vi "EstimateErrors.vi"(7 "Pose0 (X, Y, Theta)":dbl[](array[numeric])=[0.0, 0.0, 0.0], 8 "Circle variables errors":T4={"punktDistSquare"=[0.0, 0.07564773182654234, 0.07557311216319511, 0.07578803616247684, 0.07567014980458597, 0.07535518316388122, 0.0757185080544904, 0.07334892874492238, 0.07585576670877042, 0.07541545264649341, 0.07457142815247282, 0.0720824805087417, 0.06961575822916764, 0.06683871762791828, 0.0630284017195026, 0.059082964720348206, 0.05355458998235239, 0.05045461701579379, 0.04470630680818257, 0.03964739483907835, 0.03453253618111823, 0.02904994482413108, 0.023688402162769955, 0.01892536585845739, 0.014215766563588304, 0.010250329125772036, 0.006818695465891372, 0.003943465844516061, 0.0020809448605467406, 0.0005220835606117719, 1.2383649131457327e-05, 0.0003390725932862521, 0.001540945833685875, 0.0035195264049144095, 0.0060279610827917935, 0.008761138637480492, 0.012367610332300055, 0.01627487568319867, 0.020308106515570287, 0.024594534493235544, 0.028943415071940114, 0.03341115784396496, 0.037285381727813045, 0.04126201164451483, 0.045079825351421264, 0.04914306964453862, 0.0514613643484263, 0.05428534924131425, 0.05625555787449453, 0.05657242294416296, 0.05651616674073519, 0.055951366501415835, 0.054616628689924826, 0.05239466959604635, 0.05005043029476607, 0.04679005433056029, 0.042887475499745156, 0.0387519129163008, 0.0336280677551115, 0.02966200797528215, 0.025266909215039494, 0.02072471019982025, 0.016797122005156952, 0.012291220019395255, 0.008810089263448142, 0.00567593978669209, 0.003349003924343437, 0.0014861104439980038, 0.00043833446681027654, 3.9034156999441e-06, 0.00010421819224661581, 0.0006618229911799063, 0.0013807697493980796, 0.002218800940383718, 0.0032733224891644593, 0.004574912694052916, 0.005507405786350822, 0.006413953108626536, 0.007416403488251084, 0.007799062706470956, 0.007900128314354375, 0.007695822505959842, 0.007105496206833856, 0.006394343915694971, 0.005455973268666394, 0.004255972699592567, 0.0029149765928852653, 0.001966512463123503, 0.0009603861261508478, 0.0002841530345349927, 8.156616622773978e-06, 0.0004068005644318846, 0.0016844789753319045, 0.0036816048553430366, 0.007279831590487791, 0.01211319395311253, 0.018235687252944322, 0.025815049718371556, 0.03477395530382172, 0.04594658715803277, 0.05940579170402822, 0.07195291174212014, 0.08883550205094089, 0.10614135307735591, 0.12610066821536306, 0.14715212125088853, 0.1717623938366619, 0.1969362684280186, 0.2248206059063523, 0.00012726523840876527, 0.00012280960585971167, 3.0014150177905496e-05, 0.00044221993068126696, 0.0026874041910711797, 0.015825445797725355, 0.04630193476148654, 0.07938556772924259, 0.09054009974589632], "X travelled"=[0.0, 1.2695120888079892, 1.2692312255127836, 1.2694654526261373, 1.2692477473907526, 1.2691017901849175, 1.2696542995423077, 1.2571532097357658, 1.2387575500923158, 1.216600111019282, 1.192192947184398, 1.167405514173482, 1.1413899163623515, 1.1150560373224825, 1.0874230986410096, 1.0638480524217664, 1.0398001723629628, 1.0146852541804219, 0.9923351075893959, 0.9685827340265091, 0.9432369365366903, 0.9170882628506359, 0.8917289878071746, 0.8686417555900694, 0.8439669533526823, 0.8199720439623648, 0.7956956103849276, 0.7720631355922368, 0.7489369018852821, 0.7237191149505686, 0.6992024917565707, 0.6747186374632433, 0.6503530875312046, 0.6252720411425005, 0.6017948697201847, 0.5788637764853476, 0.5550605203636303, 0.5312645310848891, 0.5077586901078085, 0.48151679846144435, 0.45674499934516527, 0.42976239752787115, 0.4047903368931877, 0.37800013536527355, 0.353457975553972, 0.321633095547316, 0.29685338790972066, 0.26621470497176003, 0.23640735895233098, 0.2046386706338113, 0.1757786957333123, 0.14453904740116533, 0.11588563434771729, 0.08443371862104453, 0.0561871655388403, 0.026630408440516815, -0.00314924246510887, -0.030887936500388236, -0.06070435130947068, -0.08903243103192268, -0.11216261518885712, -0.1391091582848538, -0.1654116103393078, -0.19101893289595676, -0.2152215884303818, -0.23994715714337814, -0.265062748085184, -0.28831589903809757, -0.3118249838362658, -0.33485539410810033, -0.35943310881112206, -0.38168948393512264, -0.4051724359779647, -0.4317614148947837, -0.4544812996670769, -0.47653452740076285, -0.5026117792886527, -0.5258360330870897, -0.5507479667209695, -0.5766609558687512, -0.6002049112959483, -0.6265170935089266, -0.6519533931466335, -0.6785689453981383, -0.7034682073883944, -0.7278750721133671, -0.757191632268316, -0.7841548638522253, -0.8126279679466061, -0.8402415342318459, -0.8700108849679966, -0.9003257232864297, -0.9319275221467972, -0.9601668175409852, -0.9911787612489938, -1.0225070550459336, -1.0530758282656856, -1.0832624494521472, -1.113028095420975, -1.1441614405859464, -1.1746594514768973, -1.2021620653253586, -1.231726719500456, -1.2590665391582947, -1.2879782803828206, -1.3153404019292236, -1.3437046572531026, -1.3710522627012873, -1.398141963895538, -0.9209240462698031, -0.9210089892186536, -0.9041765205215978, -0.8566600027574827, -0.7504973452310854, -0.6062134912938122, -0.43036863858250807, -0.2550474545013706, -0.12907825402937256], "Y travelled"=[0.0, 1.2997835570201033, 1.299918266998385, 1.2995290477144008, 1.2997419532092793, 1.3003139694205859, 1.2996536097512235, 1.3039920884611322, 1.2994203274600276, 1.3002295297448985, 1.3017859072669729, 1.3063977887786817, 1.311048954293369, 1.316389275617112, 1.3238759854456834, 1.33188115664532, 1.3435550315578317, 1.3503687265675801, 1.3635524859658168, 1.375893604914819, 1.3891951203545152, 1.4045990740324474, 1.421146766916605, 1.4375053137323193, 1.4558644369719869, 1.4738853501994724, 1.4925638161546586, 1.5123376556556292, 1.5295457563837995, 1.5523340107584074, 1.5719536798753582, 1.5935114583075545, 1.6143863909036604, 1.634504558758891, 1.6528717287556438, 1.6688520864593281, 1.6864617161758972, 1.7028457289160475, 1.7178066107992285, 1.732135219670476, 1.7454546164708304, 1.758131127043267, 1.7684545144678636, 1.7785136756666506, 1.7877191136549149, 1.7970948178568789, 1.8022807728780508, 1.808436129290746, 1.8126471307419418, 1.8133410693098495, 1.8132335115605274, 1.8120709817533533, 1.8092419191532152, 1.804468328920625, 1.7992945699811371, 1.7919075661447772, 1.7827107912063302, 1.7724991714524176, 1.7590423567427707, 1.7478950251350323, 1.734648646961109, 1.7196602851886198, 1.7053321558620678, 1.6866123399737936, 1.6696203858108163, 1.651108728261376, 1.6336564904406876, 1.6142896803462332, 1.5967434706070807, 1.5774676467398316, 1.559575053267482, 1.5380139222042355, 1.5202931680977338, 1.5020652392071476, 1.4831114145715987, 1.4640399847051702, 1.44633932925363, 1.4286940336279008, 1.4100473033558134, 1.3934713992454555, 1.3785351020910583, 1.3639032285078156, 1.3508931942803428, 1.3365341066050573, 1.3256050266509627, 1.3176014816898536, 1.306502275234161, 1.2953169075402846, 1.2876909060075314, 1.2797977569282104, 1.2749442960425688, 1.2696805567666585, 1.2664096698763037, 1.2639092252393325, 1.2643295206125267, 1.2646313441406596, 1.2662172911660277, 1.2693340306245853, 1.273250028069598, 1.2786250047164172, 1.2863436394563064, 1.2893514799759693, 1.2987257080431716, 1.307715372397717, 1.3171558179397458, 1.3274743163358067, 1.3405108730642281, 1.3523620445922784, 1.366490163526435, -0.6855341381820631, -0.6857707309878518, -0.7136948176982961, -0.8033890120521333, -0.9346796502513917, -1.106006471640569, -1.2607529582490453, -1.3395413306604762, -1.358591049628456]}, 9 "Pose (X, Y, Theta)":dbl[](array[numeric])=[0.0, 0.0, 0.0], 10 "Trajectory":T6={"X path"=array[1899 elements], "Y path"=array[1899 elements], "Theta path"=array[1899 elements]}, 11 "Clear Graph":bool) -> (0 "Circle variables errors out":T5={"punktDistSquare"=[0.0+0.0i, 0.07564773182654234+0.0i, 0.07557311216319511+0.0i, 0.07578803616247684+0.0i, 0.07567014980458597+0.0i, 0.07535518316388122+0.0i, 0.0757185080544904+0.0i, 0.07334892874492238+0.0i, 0.07585576670877042+0.0i, 0.07541545264649341+0.0i, 0.07457142815247282+0.0i, 0.0720824805087417+0.0i, 0.06961575822916764+0.0i, 0.06683871762791828+0.0i, 0.0630284017195026+0.0i, 0.059082964720348206+0.0i, 0.05355458998235239+0.0i, 0.05045461701579379+0.0i, 0.04470630680818257+0.0i, 0.03964739483907835+0.0i, 0.03453253618111823+0.0i, 0.02904994482413108+0.0i, 0.023688402162769955+0.0i, 0.01892536585845739+0.0i, 0.014215766563588304+0.0i, 0.010250329125772036+0.0i, 0.006818695465891372+0.0i, 0.003943465844516061+0.0i, 0.0020809448605467406+0.0i, 0.0005220835606117719+0.0i, 1.2383649131457327e-05+0.0i, 0.0003390725932862521+0.0i, 0.001540945833685875+0.0i, 0.0035195264049144095+0.0i, 0.0060279610827917935+0.0i, 0.008761138637480492+0.0i, 0.012367610332300055+0.0i, 0.01627487568319867+0.0i, 0.020308106515570287+0.0i, 0.024594534493235544+0.0i, 0.028943415071940114+0.0i, 0.03341115784396496+0.0i, 0.037285381727813045+0.0i, 0.04126201164451483+0.0i, 0.045079825351421264+0.0i, 0.04914306964453862+0.0i, 0.0514613643484263+0.0i, 0.05428534924131425+0.0i, 0.05625555787449453+0.0i, 0.05657242294416296+0.0i, 0.05651616674073519+0.0i, 0.055951366501415835+0.0i, 0.054616628689924826+0.0i, 0.05239466959604635+0.0i, 0.05005043029476607+0.0i, 0.04679005433056029+0.0i, 0.042887475499745156+0.0i, 0.0387519129163008+0.0i, 0.0336280677551115+0.0i, 0.02966200797528215+0.0i, 0.025266909215039494+0.0i, 0.02072471019982025+0.0i, 0.016797122005156952+0.0i, 0.012291220019395255+0.0i, 0.008810089263448142+0.0i, 0.00567593978669209+0.0i, 0.003349003924343437+0.0i, 0.0014861104439980038+0.0i, 0.00043833446681027654+0.0i, 3.9034156999441e-06+0.0i, 0.00010421819224661581+0.0i, 0.0006618229911799063+0.0i, 0.0013807697493980796+0.0i, 0.002218800940383718+0.0i, 0.0032733224891644593+0.0i, 0.004574912694052916+0.0i, 0.005507405786350822+0.0i, 0.006413953108626536+0.0i, 0.007416403488251084+0.0i, 0.007799062706470956+0.0i, 0.007900128314354375+0.0i, 0.007695822505959842+0.0i, 0.007105496206833856+0.0i, 0.006394343915694971+0.0i, 0.005455973268666394+0.0i, 0.004255972699592567+0.0i, 0.0029149765928852653+0.0i, 0.001966512463123503+0.0i, 0.0009603861261508478+0.0i, 0.0002841530345349927+0.0i, 8.156616622773978e-06+0.0i, 0.0004068005644318846+0.0i, 0.0016844789753319045+0.0i, 0.0036816048553430366+0.0i, 0.007279831590487791+0.0i, 0.01211319395311253+0.0i, 0.018235687252944322+0.0i, 0.025815049718371556+0.0i, 0.03477395530382172+0.0i, 0.04594658715803277+0.0i, 0.05940579170402822+0.0i, 0.07195291174212014+0.0i, 0.08883550205094089+0.0i, 0.10614135307735591+0.0i, 0.12610066821536306+0.0i, 0.14715212125088853+0.0i, 0.1717623938366619+0.0i, 0.1969362684280186+0.0i, 0.2248206059063523+0.0i, 0.00012726523840876527+0.0i, 0.00012280960585971167+0.0i, 3.0014150177905496e-05+0.0i, 0.00044221993068126696+0.0i, 0.0026874041910711797+0.0i, 0.015825445797725355+0.0i, 0.04630193476148654+0.0i, 0.07938556772924259+0.0i, 0.09054009974589632+0.0i, 0.0887296013230938+0.0i], "TrackX"=[0.0, 1.2695120888079892, 1.2692312255127836, 1.2694654526261373, 1.2692477473907526, 1.2691017901849175, 1.2696542995423077, 1.2571532097357658, 1.2387575500923158, 1.216600111019282, 1.192192947184398, 1.167405514173482, 1.1413899163623515, 1.1150560373224825, 1.0874230986410096, 1.0638480524217664, 1.0398001723629628, 1.0146852541804219, 0.9923351075893959, 0.9685827340265091, 0.9432369365366903, 0.9170882628506359, 0.8917289878071746, 0.8686417555900694, 0.8439669533526823, 0.8199720439623648, 0.7956956103849276, 0.7720631355922368, 0.7489369018852821, 0.7237191149505686, 0.6992024917565707, 0.6747186374632433, 0.6503530875312046, 0.6252720411425005, 0.6017948697201847, 0.5788637764853476, 0.5550605203636303, 0.5312645310848891, 0.5077586901078085, 0.48151679846144435, 0.45674499934516527, 0.42976239752787115, 0.4047903368931877, 0.37800013536527355, 0.353457975553972, 0.321633095547316, 0.29685338790972066, 0.26621470497176003, 0.23640735895233098, 0.2046386706338113, 0.1757786957333123, 0.14453904740116533, 0.11588563434771729, 0.08443371862104453, 0.0561871655388403, 0.026630408440516815, -0.00314924246510887, -0.030887936500388236, -0.06070435130947068, -0.08903243103192268, -0.11216261518885712, -0.1391091582848538, -0.1654116103393078, -0.19101893289595676, -0.2152215884303818, -0.23994715714337814, -0.265062748085184, -0.28831589903809757, -0.3118249838362658, -0.33485539410810033, -0.35943310881112206, -0.38168948393512264, -0.4051724359779647, -0.4317614148947837, -0.4544812996670769, -0.47653452740076285, -0.5026117792886527, -0.5258360330870897, -0.5507479667209695, -0.5766609558687512, -0.6002049112959483, -0.6265170935089266, -0.6519533931466335, -0.6785689453981383, -0.7034682073883944, -0.7278750721133671, -0.757191632268316, -0.7841548638522253, -0.8126279679466061, -0.8402415342318459, -0.8700108849679966, -0.9003257232864297, -0.9319275221467972, -0.9601668175409852, -0.9911787612489938, -1.0225070550459336, -1.0530758282656856, -1.0832624494521472, -1.113028095420975, -1.1441614405859464, -1.1746594514768973, -1.2021620653253586, -1.231726719500456, -1.2590665391582947, -1.2879782803828206, -1.3153404019292236, -1.3437046572531026, -1.3710522627012873, -1.398141963895538, -0.9209240462698031, -0.9210089892186536, -0.9041765205215978, -0.8566600027574827, -0.7504973452310854, -0.6062134912938122, -0.43036863858250807, -0.2550474545013706, -0.12907825402937256, -0.06378735155907347], "TrackY"=[0.0, 1.2997835570201033, 1.299918266998385, 1.2995290477144008, 1.2997419532092793, 1.3003139694205859, 1.2996536097512235, 1.3039920884611322, 1.2994203274600276, 1.3002295297448985, 1.3017859072669729, 1.3063977887786817, 1.311048954293369, 1.316389275617112, 1.3238759854456834, 1.33188115664532, 1.3435550315578317, 1.3503687265675801, 1.3635524859658168, 1.375893604914819, 1.3891951203545152, 1.4045990740324474, 1.421146766916605, 1.4375053137323193, 1.4558644369719869, 1.4738853501994724, 1.4925638161546586, 1.5123376556556292, 1.5295457563837995, 1.5523340107584074, 1.5719536798753582, 1.5935114583075545, 1.6143863909036604, 1.634504558758891, 1.6528717287556438, 1.6688520864593281, 1.6864617161758972, 1.7028457289160475, 1.7178066107992285, 1.732135219670476, 1.7454546164708304, 1.758131127043267, 1.7684545144678636, 1.7785136756666506, 1.7877191136549149, 1.7970948178568789, 1.8022807728780508, 1.808436129290746, 1.8126471307419418, 1.8133410693098495, 1.8132335115605274, 1.8120709817533533, 1.8092419191532152, 1.804468328920625, 1.7992945699811371, 1.7919075661447772, 1.7827107912063302, 1.7724991714524176, 1.7590423567427707, 1.7478950251350323, 1.734648646961109, 1.7196602851886198, 1.7053321558620678, 1.6866123399737936, 1.6696203858108163, 1.651108728261376, 1.6336564904406876, 1.6142896803462332, 1.5967434706070807, 1.5774676467398316, 1.559575053267482, 1.5380139222042355, 1.5202931680977338, 1.5020652392071476, 1.4831114145715987, 1.4640399847051702, 1.44633932925363, 1.4286940336279008, 1.4100473033558134, 1.3934713992454555, 1.3785351020910583, 1.3639032285078156, 1.3508931942803428, 1.3365341066050573, 1.3256050266509627, 1.3176014816898536, 1.306502275234161, 1.2953169075402846, 1.2876909060075314, 1.2797977569282104, 1.2749442960425688, 1.2696805567666585, 1.2664096698763037, 1.2639092252393325, 1.2643295206125267, 1.2646313441406596, 1.2662172911660277, 1.2693340306245853, 1.273250028069598, 1.2786250047164172, 1.2863436394563064, 1.2893514799759693, 1.2987257080431716, 1.307715372397717, 1.3171558179397458, 1.3274743163358067, 1.3405108730642281, 1.3523620445922784, 1.366490163526435, -0.6855341381820631, -0.6857707309878518, -0.7136948176982961, -0.8033890120521333, -0.9346796502513917, -1.106006471640569, -1.2607529582490453, -1.3395413306604762, -1.358591049628456, -1.3555183923263967]}, 1 "PathController inputs":T1, 2 "Truck data":T2={"RMS error"=0.0+0.0i, "DistanceAheadPointToTrajectory"=0.0+0.0i, "CurrentRefTheta"=0.04056520868612421, "CurrentThetaError"=-6.222088142143954, "DistanceCurrentPoseToTrajectory"=0.29787514384905267+0.0i, "MaximalDistance"=0.4741525133396978+0.0i}, 4 "Errors":cluster{"error_x":dbl, "error_y":dbl}, 5 "Plot variables":T3={"currentRefX"=-0.06646440361680006, "currentRefY"=-1.05765527827, "pointAhead"=[-0.06378735155907347, -1.3555183923263967], "TrackX"=[0.0, 1.2695120888079892, 1.2692312255127836, 1.2694654526261373, 1.2692477473907526, 1.2691017901849175, 1.2696542995423077, 1.2571532097357658, 1.2387575500923158, 1.216600111019282, 1.192192947184398, 1.167405514173482, 1.1413899163623515, 1.1150560373224825, 1.0874230986410096, 1.0638480524217664, 1.0398001723629628, 1.0146852541804219, 0.9923351075893959, 0.9685827340265091, 0.9432369365366903, 0.9170882628506359, 0.8917289878071746, 0.8686417555900694, 0.8439669533526823, 0.8199720439623648, 0.7956956103849276, 0.7720631355922368, 0.7489369018852821, 0.7237191149505686, 0.6992024917565707, 0.6747186374632433, 0.6503530875312046, 0.6252720411425005, 0.6017948697201847, 0.5788637764853476, 0.5550605203636303, 0.5312645310848891, 0.5077586901078085, 0.48151679846144435, 0.45674499934516527, 0.42976239752787115, 0.4047903368931877, 0.37800013536527355, 0.353457975553972, 0.321633095547316, 0.29685338790972066, 0.26621470497176003, 0.23640735895233098, 0.2046386706338113, 0.1757786957333123, 0.14453904740116533, 0.11588563434771729, 0.08443371862104453, 0.0561871655388403, 0.026630408440516815, -0.00314924246510887, -0.030887936500388236, -0.06070435130947068, -0.08903243103192268, -0.11216261518885712, -0.1391091582848538, -0.1654116103393078, -0.19101893289595676, -0.2152215884303818, -0.23994715714337814, -0.265062748085184, -0.28831589903809757, -0.3118249838362658, -0.33485539410810033, -0.35943310881112206, -0.38168948393512264, -0.4051724359779647, -0.4317614148947837, -0.4544812996670769, -0.47653452740076285, -0.5026117792886527, -0.5258360330870897, -0.5507479667209695, -0.5766609558687512, -0.6002049112959483, -0.6265170935089266, -0.6519533931466335, -0.6785689453981383, -0.7034682073883944, -0.7278750721133671, -0.757191632268316, -0.7841548638522253, -0.8126279679466061, -0.8402415342318459, -0.8700108849679966, -0.9003257232864297, -0.9319275221467972, -0.9601668175409852, -0.9911787612489938, -1.0225070550459336, -1.0530758282656856, -1.0832624494521472, -1.113028095420975, -1.1441614405859464, -1.1746594514768973, -1.2021620653253586, -1.231726719500456, -1.2590665391582947, -1.2879782803828206, -1.3153404019292236, -1.3437046572531026, -1.3710522627012873, -1.398141963895538, -0.9209240462698031, -0.9210089892186536, -0.9041765205215978, -0.8566600027574827, -0.7504973452310854, -0.6062134912938122, -0.43036863858250807, -0.2550474545013706, -0.12907825402937256, -0.06378735155907347], "TrackY"=[0.0, 1.2997835570201033, 1.299918266998385, 1.2995290477144008, 1.2997419532092793, 1.3003139694205859, 1.2996536097512235, 1.3039920884611322, 1.2994203274600276, 1.3002295297448985, 1.3017859072669729, 1.3063977887786817, 1.311048954293369, 1.316389275617112, 1.3238759854456834, 1.33188115664532, 1.3435550315578317, 1.3503687265675801, 1.3635524859658168, 1.375893604914819, 1.3891951203545152, 1.4045990740324474, 1.421146766916605, 1.4375053137323193, 1.4558644369719869, 1.4738853501994724, 1.4925638161546586, 1.5123376556556292, 1.5295457563837995, 1.5523340107584074, 1.5719536798753582, 1.5935114583075545, 1.6143863909036604, 1.634504558758891, 1.6528717287556438, 1.6688520864593281, 1.6864617161758972, 1.7028457289160475, 1.7178066107992285, 1.732135219670476, 1.7454546164708304, 1.758131127043267, 1.7684545144678636, 1.7785136756666506, 1.7877191136549149, 1.7970948178568789, 1.8022807728780508, 1.808436129290746, 1.8126471307419418, 1.8133410693098495, 1.8132335115605274, 1.8120709817533533, 1.8092419191532152, 1.804468328920625, 1.7992945699811371, 1.7919075661447772, 1.7827107912063302, 1.7724991714524176, 1.7590423567427707, 1.7478950251350323, 1.734648646961109, 1.7196602851886198, 1.7053321558620678, 1.6866123399737936, 1.6696203858108163, 1.651108728261376, 1.6336564904406876, 1.6142896803462332, 1.5967434706070807, 1.5774676467398316, 1.559575053267482, 1.5380139222042355, 1.5202931680977338, 1.5020652392071476, 1.4831114145715987, 1.4640399847051702, 1.44633932925363, 1.4286940336279008, 1.4100473033558134, 1.3934713992454555, 1.3785351020910583, 1.3639032285078156, 1.3508931942803428, 1.3365341066050573, 1.3256050266509627, 1.3176014816898536, 1.306502275234161, 1.2953169075402846, 1.2876909060075314, 1.2797977569282104, 1.2749442960425688, 1.2696805567666585, 1.2664096698763037, 1.2639092252393325, 1.2643295206125267, 1.2646313441406596, 1.2662172911660277, 1.2693340306245853, 1.273250028069598, 1.2786250047164172, 1.2863436394563064, 1.2893514799759693, 1.2987257080431716, 1.307715372397717, 1.3171558179397458, 1.3274743163358067, 1.3405108730642281, 1.3523620445922784, 1.366490163526435, -0.6855341381820631, -0.6857707309878518, -0.7136948176982961, -0.8033890120521333, -0.9346796502513917, -1.106006471640569, -1.2607529582490453, -1.3395413306604762, -1.358591049628456, -1.3555183923263967]})   [LabVIEW 2013]
uses:
  <vilib>/imath/engines/lvmath2/RunTimeEngine/ErrorHandling/NIMS_Finalize Error.vi
  <vilib>/imath/engines/lvmath2/RunTimeEngine/Managers/WorkSpace/UID Generator.vi
  <vilib>/imath/engines/lvmath2/RunTimeEngine/IndexRead/NIMS V(S).vi
  <instcachedir>/0/NIMS V(S)_0488751826AF41519A22953C041130DC.lvgen/NIMS V(S)_0488751826AF41519A22953C041130DC_000.vi
  <vilib>/imath/engines/lvmath2/RunTimeEngine/BuiltInFunctions/is_nan/NIMS_is_nan.vi
  <instcachedir>/0/NIMS_is_nan_BCCD798162CC49E3A8E57072444F6EB6.lvgen/NIMS_is_nan_BCCD798162CC49E3A8E57072444F6EB6_002.vi
  <vilib>/imathl/engines/lvmath/Functions/Error Handling/Create Error.vi
  <vilib>/imath/engines/lvmath2/RunTimeEngine/Managers/SymbolTable/Clear UID.vi
  <vilib>/imath/engines/lvmath2/RunTimeEngine/NodeEndStatement/NIMS_NodeEndStatement_Output.vi
  <instcachedir>/0/NIMS_NodeEndStatement_Output_53EC0D466D134D7ABD903AC30B43404B.lvgen/NIMS_NodeEndStatement_Output_53EC0D466D134D7ABD903AC30B43404B_010.vi
  <instcachedir>/0/NIMS_NodeEndStatement_Output_53EC0D466D134D7ABD903AC30B43404B.lvgen/NIMS_NodeEndStatement_Output_53EC0D466D134D7ABD903AC30B43404B_001.vi
  <instcachedir>/0/NIMS_NodeEndStatement_Output_53EC0D466D134D7ABD903AC30B43404B.lvgen/NIMS_NodeEndStatement_Output_53EC0D466D134D7ABD903AC30B43404B_009.vi
  <instcachedir>/0/NIMS_NodeEndStatement_Output_53EC0D466D134D7ABD903AC30B43404B.lvgen/NIMS_NodeEndStatement_Output_53EC0D466D134D7ABD903AC30B43404B_005.vi
  <instcachedir>/0/NIMS_NodeEndStatement_Output_53EC0D466D134D7ABD903AC30B43404B.lvgen/NIMS_NodeEndStatement_Output_53EC0D466D134D7ABD903AC30B43404B_000.vi
  <vilib>/imath/engines/lvmath2/RunTimeEngine/IndexRead/NIMS V(R2).vi
  <instcachedir>/0/NIMS V(R2)_C76619605A0E4E9F8B2FA9389712AC47.lvgen/NIMS V(R2)_C76619605A0E4E9F8B2FA9389712AC47_000.vi
  <vilib>/imath/engines/lvmath2/RunTimeEngine/ArithmeticOperatorToken/NIMS_ArithmeticOperator_plus.vi
  <instcachedir>/0/NIMS_ArithmeticOperator_plus_8A46DAFC24D445C9B2C97B626139369E.lvgen/NIMS_ArithmeticOperator_plus_8A46DAFC24D445C9B2C97B626139369E_004.vi
  <vilib>/imath/engines/lvmath2/RunTimeEngine/RunTimeType/NIMS_RunTimeType_From StrictType (excl LVString).vi
  <instcachedir>/0/NIMS_RunTimeType_From StrictType (excl LVString)_4DEE718D6EB74582AA20236969C084FC.lvgen/NIMS_RunTimeType_From StrictType (excl LVString)_4DEE718D6EB74582AA20236969C084FC_000.vi
  <vilib>/imath/engines/lvmath2/RunTimeEngine/LocalVariableDefStatement/MC_LocalVariableDefStatement_Display.vi
  <vilib>/imath/engines/lvmath2/RunTimeEngine/ErrorHandling/NIMS_Create Error From Enums.vi
  <vilib>/imath/engines/lvmath2/RunTimeEngine/BuiltInFunctions/min/1 input/NIMS_min(CV).vi
  <instcachedir>/0/NIMS_min(CV)_46E60952406B4159AB512BDF500C959F.lvgen/NIMS_min(CV)_46E60952406B4159AB512BDF500C959F_000.vi
  <vilib>/imath/engines/lvmath2/RunTimeEngine/ArithmeticOperatorToken/NIMS_ArithmeticOperator_power(S).vi
  <instcachedir>/0/NIMS_ArithmeticOperator_power(S)_7602F12E697C47D8910FAD43BB85D848.lvgen/NIMS_ArithmeticOperator_power(S)_7602F12E697C47D8910FAD43BB85D848_010.vi
  <vilib>/imath/engines/lvmath2/RunTimeEngine/BuiltInFunctions/length/NIMS_length(GV).vi
  <instcachedir>/0/NIMS_length(GV)_08A3D13377FD4E4B96F5795FBF3698FA.lvgen/NIMS_length(GV)_08A3D13377FD4E4B96F5795FBF3698FA_001.vi
  <vilib>/imath/engines/lvmath2/RunTimeEngine/BuiltInFunctions/sum/NIMS_sum(GV).vi
  <instcachedir>/0/NIMS_sum(GV)_67F5EC36BC034E54A6BEC5B0673C00E5.lvgen/NIMS_sum(GV)_67F5EC36BC034E54A6BEC5B0673C00E5_001.vi
  <vilib>/imath/engines/lvmath2/RunTimeEngine/BuiltInFunctions/max/1 input/NIMS_max(CV).vi
  <instcachedir>/0/NIMS_max(CV)_CD1B6316A64149E4A502EA6FA3107FD7.lvgen/NIMS_max(CV)_CD1B6316A64149E4A502EA6FA3107FD7_000.vi
  <vilib>/imath/engines/lvmath2/RunTimeEngine/Managers/SymbolTable/NIMS_WorkSpace.lvlib
panel:
  out "hejsan":i32
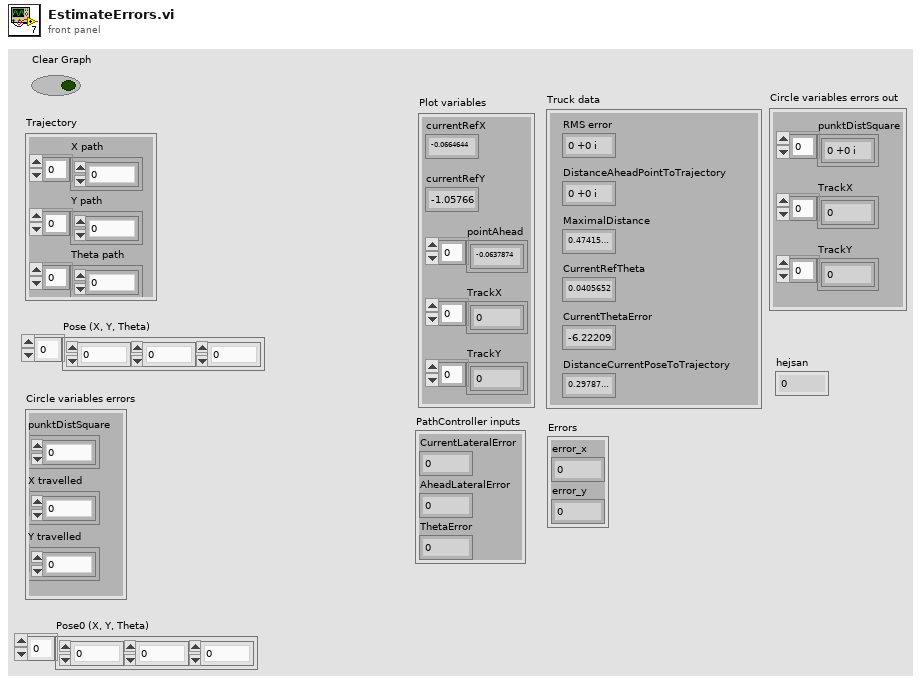
[diagram p1: front panel]
types:
  T1 = cluster{"CurrentLateralError":dbl, "AheadLateralError":dbl, "ThetaError":dbl}
  T2 = cluster{"RMS error":cdb, "DistanceAheadPointToTrajectory":cdb, "CurrentRefTheta":dbl, "CurrentThetaError":dbl, "DistanceCurrentPoseToTrajectory":cdb, "MaximalDistance":cdb}
  T3 = cluster{"currentRefX":dbl, "currentRefY":dbl, "pointAhead":dbl[], "TrackX":dbl[], "TrackY":dbl[]}
  T4 = cluster{"punktDistSquare":dbl[], "X travelled":dbl[], "Y travelled":dbl[]}
  T5 = cluster{"punktDistSquare":cdb[], "TrackX":dbl[], "TrackY":dbl[]}
  T6 = cluster{"X path":dbl[], "Y path":dbl[], "Theta path":dbl[]}
  T7 = cluster{"rms":cdb, "close":cdb, "currentRefTheta":dbl, "e_theta_closest":dbl, "punktDist":cdb, "distMax":cdb}
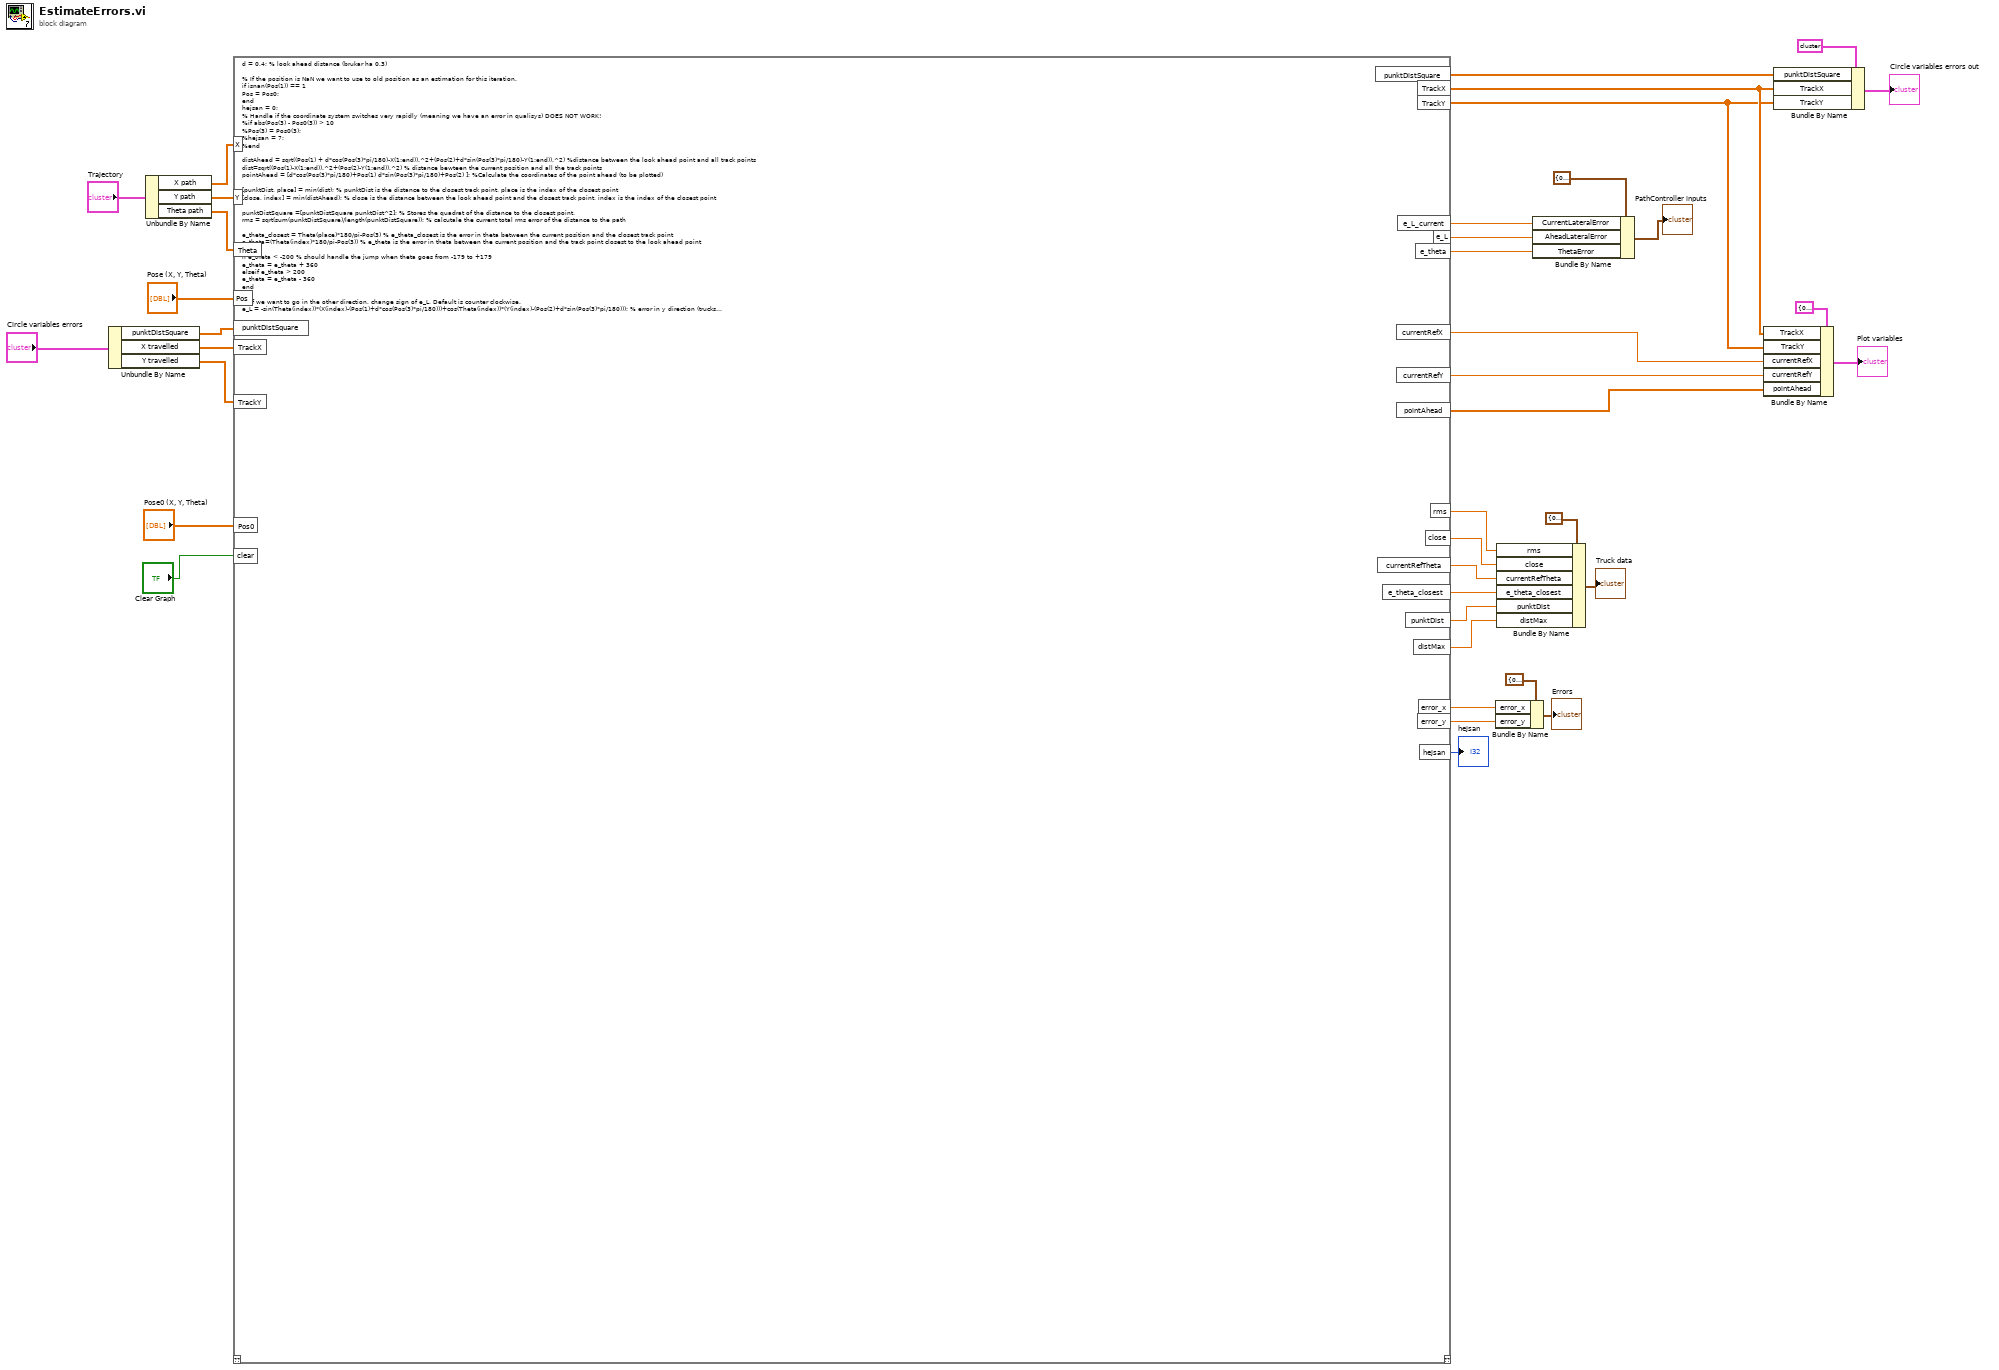
[diagram p0: block diagram]
diagram:
  n1 = Unbundle By Name("Circle variables errors") -> ("punktDistSquare"=w31:dbl[], "X travelled"=w32:dbl[], "Y travelled"=w33:dbl[])
  n2 = Unbundle By Name("Trajectory") -> ("X path"=w37:dbl[], "Y path"=w36:dbl[], "Theta path"=w35:dbl[])
  n3 = mathscript code="d = 0.4; % look ahead distance (brukar ha 0.3)\n\n% If the position is NaN we want to use to old position as an estimation for this iteration.\nif isnan(Pos(1)) == 1\nPos = Pos0;\nend\nhejsan = 0;\n% Handle if the coordinate system switches very rapidly (meaning we have an error in qualisys) DOES NOT WORK!\n%if abs(Pos(3) - Pos0(3)) > 10\n%Pos(3) = Pos0(3);\n%hejsan = 7;\n%end\n\ndistAhead = sqrt((Pos(1) + d*cos(Pos(3)*pi/180)-X(1:end)).^2+(Pos(2)+d*sin(Pos(3)*pi/180)-Y(1:end)).^2) %distance between the look ahead point and all track points\ndist=sqrt((Pos(1)-X(1:end)).^2+(Pos(2)-Y(1:end)).^2) % distance bewteen the current position and all the track points\npointAhead = [d*cos(Pos(3)*pi/180)+Pos(1) d*sin(Pos(3)*pi/180)+Pos(2) ]; %Calculate the coordinates of the point ahead (to be plotted)\n\n[punktDist, place] = min(dist); % punktDist is the distance to the closest track point, place is the index of the closest point\n[close, index] = min(distAhead); % close is the distance between the look ahead point and the closest track point, index is the index of the closest point\n\npunktDistSquare =[punktDistSquare punktDist^2]; % Stores the quadrat of the distance to the closest point.\nrms = sqrt(sum(punktDistSquare)/length(punktDistSquare)); % calcutale the current total rms error of the distance to the path\n\ne_theta_closest = Theta(place)*180/pi-Pos(3) % e_theta_closest is the error in theta between the current position and the closest track point\ne_theta=(Theta(index)*180/pi-Pos(3)) % e_theta is the error in theta between the current position and the track point closest to the look ahead point\n\nif e_theta < -200 % should handle the jump when theta goes from -179 to +179\ne_theta = e_theta + 360\nelseif e_theta > 200\ne_theta = e_theta - 360 \nend\n\n% If we want to go in the other direction, change sign of e_L. Default is counter clockwise.\ne_L = -sin(Theta(index))*(X(index)-(Pos(1)+d*cos(Pos(3)*pi/180)))+cos(Theta(index))*(Y(index)-(Pos(2)+d*sin(Pos(3)*pi/180))); % error in y direction (trucks coordinates) between the look ahead distance and the reference point\ne_L_current = -sin(Theta(place))*(X(place)-Pos(1))+cos(Theta(place))*(Y(place)-Pos(2)); % error in y direction (trucks coordinates) between the look ahead distance and the reference point\n\n% Defines the coordinates of the current ref. point to plot later\ncurrentRefX = X(index)\ncurrentRefY = Y(index)\ncurrentRefTheta = Theta(index)*180/pi\n\n% Gets the maximal distance to the trajectory for this run of the main program\npunktDistVector = sqrt(punktDistSquare);\ndistMax = max(punktDistVector);\n\n% Calculate errors in x and y to show\nerror_x = X(place) - Pos(1);\nerror_y = Y(place) - Pos(2);\n\n% If we press clear graph, the travelled path of the truck is set to onlythe current position. Otherwise we store the position for each iteration and plots the path.\nif clear == 1\nTrackX = [Pos(1)]\nTrackY = [Pos(2)]\nelse\nTrackX = [TrackX Pos(1)]; \nTrackY = [TrackY Pos(2)];\nend"("punktDistSquare"=w31, "X"=w37, "Y"=w36, "Theta"=w35, "Pos"="Pose (X, Y, Theta)", "TrackX"=w32, "TrackY"=w33, "Pos0"="Pose0 (X, Y, Theta)", "clear"="Clear Graph") -> ("punktDistSquare"=w4:cdb[], "TrackX"=w3:dbl[], "TrackY"=w2:dbl[], "rms"=w29:cdb, "e_L"=w9:dbl, "close"=w28:cdb, "currentRefX"=w20:dbl, "currentRefY"=w19:dbl, "currentRefTheta"=w27:dbl, "e_theta"=w8:dbl, "e_theta_closest"=w26:dbl, "punktDist"=w25:cdb, "pointAhead"=w18:dbl[], "distMax"=w24:cdb, "e_L_current"=w10:dbl, "error_x"=w17:dbl, "error_y"=w15:dbl, "hejsan"=→"hejsan":i32)  [unwired: 1 in, 1 out]
  n4 = Bundle By Name(cluster=cluster{"error_y":dbl, "error_x":dbl} {"error_y"=0.0, "error_x"=0.0} ("input cluster"), "error_x"=w17, "error_y"=w15) -> (→"Errors":cluster{"error_y":dbl, "error_x":dbl})
  n5 = Bundle By Name(cluster=T7 {"rms"=0.0+0.0i, "close"=0.0+0.0i, "currentRefTheta"=0.0, "e_theta_closest"=0.0, "punktDist"=0.0+0.0i, "distMax"=0.0+0.0i} ("Cluster 6"), "rms"=w29, "close"=w28, "currentRefTheta"=w27, "e_theta_closest"=w26, "punktDist"=w25, "distMax"=w24) -> (→"Truck data":T7)
  n6 = Bundle By Name(cluster=T1 {"CurrentLateralError"=0.0, "AheadLateralError"=0.0, "ThetaError"=0.0} ("PathController inputs"), "CurrentLateralError"=w10, "AheadLateralError"=w9, "ThetaError"=w8) -> (→"PathController inputs":T1)
  n7 = Bundle By Name(cluster=T3 {"currentRefX"=0.0, "currentRefY"=0.0, "pointAhead"=[], "TrackX"=[], "TrackY"=[]} ("Plot variables"), "TrackX"=w3, "TrackY"=w2, "currentRefX"=w20, "currentRefY"=w19, "pointAhead"=w18) -> (→"Plot variables":T3)
  n8 = Bundle By Name(cluster=T5 {"punktDistSquare"=[0.0+0.0i, 0.07564773182654234+0.0i, 0.07557311216319511+0.0i, 0.07578803616247684+0.0i, 0.07567014980458597+0.0i, 0.07535518316388122+0.0i, 0.0757185080544904+0.0i, 0.07334892874492238+0.0i, 0.07585576670877042+0.0i, 0.07541545264649341+0.0i, 0.07457142815247282+0.0i, 0.0720824805087417+0.0i, 0.06961575822916764+0.0i, 0.06683871762791828+0.0i, 0.0630284017195026+0.0i, 0.059082964720348206+0.0i, 0.05355458998235239+0.0i, 0.05045461701579379+0.0i, 0.04470630680818257+0.0i, 0.03964739483907835+0.0i, 0.03453253618111823+0.0i, 0.02904994482413108+0.0i, 0.023688402162769955+0.0i, 0.01892536585845739+0.0i, 0.014215766563588304+0.0i, 0.010250329125772036+0.0i, 0.006818695465891372+0.0i, 0.003943465844516061+0.0i, 0.0020809448605467406+0.0i, 0.0005220835606117719+0.0i, 1.2383649131457327e-05+0.0i, 0.0003390725932862521+0.0i, 0.001540945833685875+0.0i, 0.0035195264049144095+0.0i, 0.0060279610827917935+0.0i, 0.008761138637480492+0.0i, 0.012367610332300055+0.0i, 0.01627487568319867+0.0i, 0.020308106515570287+0.0i, 0.024594534493235544+0.0i, 0.028943415071940114+0.0i, 0.03341115784396496+0.0i, 0.037285381727813045+0.0i, 0.04126201164451483+0.0i, 0.045079825351421264+0.0i, 0.04914306964453862+0.0i, 0.0514613643484263+0.0i, 0.05428534924131425+0.0i, 0.05625555787449453+0.0i, 0.05657242294416296+0.0i, 0.05651616674073519+0.0i, 0.055951366501415835+0.0i, 0.054616628689924826+0.0i, 0.05239466959604635+0.0i, 0.05005043029476607+0.0i, 0.04679005433056029+0.0i, 0.042887475499745156+0.0i, 0.0387519129163008+0.0i, 0.0336280677551115+0.0i, 0.02966200797528215+0.0i, 0.025266909215039494+0.0i, 0.02072471019982025+0.0i, 0.016797122005156952+0.0i, 0.012291220019395255+0.0i, 0.008810089263448142+0.0i, 0.00567593978669209+0.0i, 0.003349003924343437+0.0i, 0.0014861104439980038+0.0i, 0.00043833446681027654+0.0i, 3.9034156999441e-06+0.0i, 0.00010421819224661581+0.0i, 0.0006618229911799063+0.0i, 0.0013807697493980796+0.0i, 0.002218800940383718+0.0i, 0.0032733224891644593+0.0i, 0.004574912694052916+0.0i, 0.005507405786350822+0.0i, 0.006413953108626536+0.0i, 0.007416403488251084+0.0i, 0.007799062706470956+0.0i, 0.007900128314354375+0.0i, 0.007695822505959842+0.0i, 0.007105496206833856+0.0i, 0.006394343915694971+0.0i, 0.005455973268666394+0.0i, 0.004255972699592567+0.0i, 0.0029149765928852653+0.0i, 0.001966512463123503+0.0i, 0.0009603861261508478+0.0i, 0.0002841530345349927+0.0i, 8.156616622773978e-06+0.0i, 0.0004068005644318846+0.0i, 0.0016844789753319045+0.0i, 0.0036816048553430366+0.0i, 0.007279831590487791+0.0i, 0.01211319395311253+0.0i, 0.018235687252944322+0.0i, 0.025815049718371556+0.0i, 0.03477395530382172+0.0i, 0.04594658715803277+0.0i, 0.05940579170402822+0.0i, 0.07195291174212014+0.0i, 0.08883550205094089+0.0i, 0.10614135307735591+0.0i, 0.12610066821536306+0.0i, 0.14715212125088853+0.0i, 0.1717623938366619+0.0i, 0.1969362684280186+0.0i, 0.2248206059063523+0.0i, 0.2509848111802271+0.0i], "TrackX"=[1.2694032014006624, 1.2695120888079892, 1.2692312255127836, 1.2694654526261373, 1.2692477473907526, 1.2691017901849175, 1.2696542995423077, 1.2571532097357658, 1.2387575500923158, 1.216600111019282, 1.192192947184398, 1.167405514173482, 1.1413899163623515, 1.1150560373224825, 1.0874230986410096, 1.0638480524217664, 1.0398001723629628, 1.0146852541804219, 0.9923351075893959, 0.9685827340265091, 0.9432369365366903, 0.9170882628506359, 0.8917289878071746, 0.8686417555900694, 0.8439669533526823, 0.8199720439623648, 0.7956956103849276, 0.7720631355922368, 0.7489369018852821, 0.7237191149505686, 0.6992024917565707, 0.6747186374632433, 0.6503530875312046, 0.6252720411425005, 0.6017948697201847, 0.5788637764853476, 0.5550605203636303, 0.5312645310848891, 0.5077586901078085, 0.48151679846144435, 0.45674499934516527, 0.42976239752787115, 0.4047903368931877, 0.37800013536527355, 0.353457975553972, 0.321633095547316, 0.29685338790972066, 0.26621470497176003, 0.23640735895233098, 0.2046386706338113, 0.1757786957333123, 0.14453904740116533, 0.11588563434771729, 0.08443371862104453, 0.0561871655388403, 0.026630408440516815, -0.00314924246510887, -0.030887936500388236, -0.06070435130947068, -0.08903243103192268, -0.11216261518885712, -0.1391091582848538, -0.1654116103393078, -0.19101893289595676, -0.2152215884303818, -0.23994715714337814, -0.265062748085184, -0.28831589903809757, -0.3118249838362658, -0.33485539410810033, -0.35943310881112206, -0.38168948393512264, -0.4051724359779647, -0.4317614148947837, -0.4544812996670769, -0.47653452740076285, -0.5026117792886527, -0.5258360330870897, -0.5507479667209695, -0.5766609558687512, -0.6002049112959483, -0.6265170935089266, -0.6519533931466335, -0.6785689453981383, -0.7034682073883944, -0.7278750721133671, -0.757191632268316, -0.7841548638522253, -0.8126279679466061, -0.8402415342318459, -0.8700108849679966, -0.9003257232864297, -0.9319275221467972, -0.9601668175409852, -0.9911787612489938, -1.0225070550459336, -1.0530758282656856, -1.0832624494521472, -1.113028095420975, -1.1441614405859464, -1.1746594514768973, -1.2021620653253586, -1.231726719500456, -1.2590665391582947, -1.2879782803828206, -1.3153404019292236, -1.3437046572531026, -1.3710522627012873, -1.398141963895538, -1.4220196882676213], "TrackY"=[1.2999333348609878, 1.2997835570201033, 1.299918266998385, 1.2995290477144008, 1.2997419532092793, 1.3003139694205859, 1.2996536097512235, 1.3039920884611322, 1.2994203274600276, 1.3002295297448985, 1.3017859072669729, 1.3063977887786817, 1.311048954293369, 1.316389275617112, 1.3238759854456834, 1.33188115664532, 1.3435550315578317, 1.3503687265675801, 1.3635524859658168, 1.375893604914819, 1.3891951203545152, 1.4045990740324474, 1.421146766916605, 1.4375053137323193, 1.4558644369719869, 1.4738853501994724, 1.4925638161546586, 1.5123376556556292, 1.5295457563837995, 1.5523340107584074, 1.5719536798753582, 1.5935114583075545, 1.6143863909036604, 1.634504558758891, 1.6528717287556438, 1.6688520864593281, 1.6864617161758972, 1.7028457289160475, 1.7178066107992285, 1.732135219670476, 1.7454546164708304, 1.758131127043267, 1.7684545144678636, 1.7785136756666506, 1.7877191136549149, 1.7970948178568789, 1.8022807728780508, 1.808436129290746, 1.8126471307419418, 1.8133410693098495, 1.8132335115605274, 1.8120709817533533, 1.8092419191532152, 1.804468328920625, 1.7992945699811371, 1.7919075661447772, 1.7827107912063302, 1.7724991714524176, 1.7590423567427707, 1.7478950251350323, 1.734648646961109, 1.7196602851886198, 1.7053321558620678, 1.6866123399737936, 1.6696203858108163, 1.651108728261376, 1.6336564904406876, 1.6142896803462332, 1.5967434706070807, 1.5774676467398316, 1.559575053267482, 1.5380139222042355, 1.5202931680977338, 1.5020652392071476, 1.4831114145715987, 1.4640399847051702, 1.44633932925363, 1.4286940336279008, 1.4100473033558134, 1.3934713992454555, 1.3785351020910583, 1.3639032285078156, 1.3508931942803428, 1.3365341066050573, 1.3256050266509627, 1.3176014816898536, 1.306502275234161, 1.2953169075402846, 1.2876909060075314, 1.2797977569282104, 1.2749442960425688, 1.2696805567666585, 1.2664096698763037, 1.2639092252393325, 1.2643295206125267, 1.2646313441406596, 1.2662172911660277, 1.2693340306245853, 1.273250028069598, 1.2786250047164172, 1.2863436394563064, 1.2893514799759693, 1.2987257080431716, 1.307715372397717, 1.3171558179397458, 1.3274743163358067, 1.3405108730642281, 1.3523620445922784, 1.366490163526435, 1.3790297556220699]} ("Circle variables"), "punktDistSquare"=w4, "TrackX"=w3, "TrackY"=w2) -> (→"Circle variables errors out":T5)
